vi "SetGlobalVariables.vi"   [LabVIEW 2023]
doc: "This VI sets non-robot specific constants and initializes critical global variables."
uses:
  GlobalMiscellaneous.vi
  GlobalDrivebase.vi
  GlobalPoseAndTargeting.vi
  GlobalShooter.vi
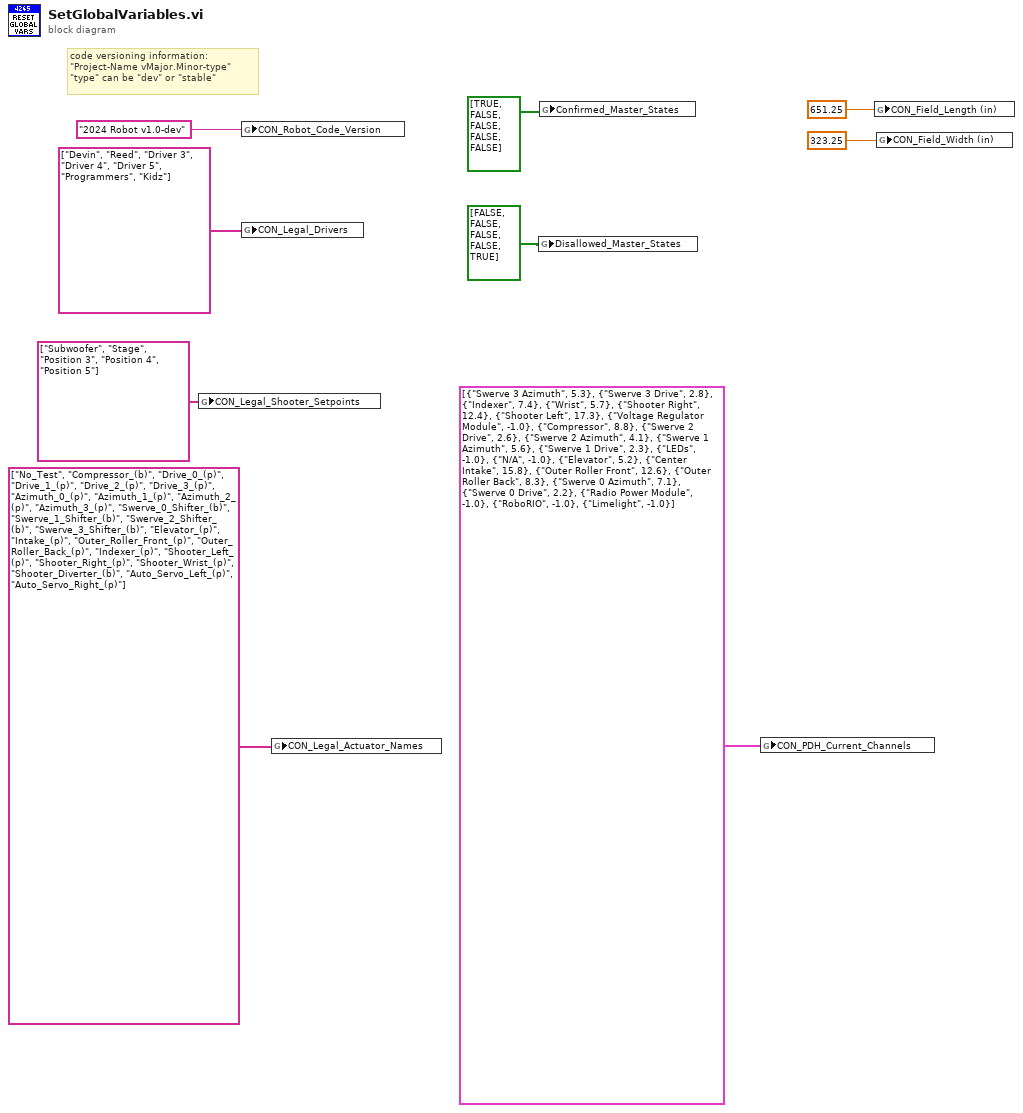
[diagram p0: block diagram]
diagram:
  # "code versioning information:\n\"Project-Name vMajor.Minor-type\"\n\"type\" can be \"dev\" or \"stable\""
  n1 = global write "GlobalShooter.vi" "CON_Legal_Shooter_Setpoints"(string[] ["Subwoofer", "Stage", "Position 3", "Position 4", "Position 5"] ("appended array")) -> ()
  n2 = global write "GlobalMiscellaneous.vi" "CON_Robot_Code_Version"("2024 Robot v1.0-dev" ("CON_Robot_Code_Version")) -> ()
  n3 = global write "GlobalDrivebase.vi" "CON_Legal_Drivers"(string[] ["Devin", "Reed", "Driver 3", "Driver 4", "Driver 5", "Programmers", "Kidz"] ("appended array")) -> ()
  n4 = global write "GlobalMiscellaneous.vi" "CON_Legal_Actuator_Names"(string[] ["No_Test", "Compressor_(b)", "Drive_0_(p)", "Drive_1_(p)", "Drive_2_(p)", "Drive_3_(p)", "Azimuth_0_(p)", "Azimuth_1_(p)", "Azimuth_2_(p)", "Azimuth_3_(p)", "Swerve_0_Shifter_(b)", "Swerve_1_Shifter_(b)", "Swerve_2_Shifter_(b)", "Swerve_3_Shifter_(b)", "Elevator_(p)", "Intake_(p)", "Outer_Roller_Front_(p)", "Outer_Roller_Back_(p)", "Indexer_(p)", "Shooter_Left_(p)", "Shooter_Right_(p)", "Shooter_Wrist_(p)", "Shooter_Diverter_(b)", "Auto_Servo_Left_(p)", "Auto_Servo_Right_(p)"] ("appended array")) -> ()
  n5 = global write "GlobalMiscellaneous.vi" "Disallowed_Master_States"(bool[] [FALSE, FALSE, FALSE, FALSE, TRUE] ("Disallowed_Master_States")) -> ()
  n6 = global write "GlobalMiscellaneous.vi" "Confirmed_Master_States"(bool[] [TRUE, FALSE, FALSE, FALSE, FALSE] ("Disallowed_Master_States")) -> ()
  n7 = global write "GlobalMiscellaneous.vi" "CON_PDH_Current_Channels"(cluster{string, dbl}[] [{"Swerve 3 Azimuth", 5.3}, {"Swerve 3 Drive", 2.8}, {"Indexer", 7.4}, {"Wrist", 5.7}, {"Shooter Right", 12.4}, {"Shooter Left", 17.3}, {"Voltage Regulator Module", -1.0}, {"Compressor", 8.8}, {"Swerve 2 Drive", 2.6}, {"Swerve 2 Azimuth", 4.1}, {"Swerve 1 Azimuth", 5.6}, {"Swerve 1 Drive", 2.3}, {"LEDs", -1.0}, {"N/A", -1.0}, {"Elevator", 5.2}, {"Center Intake", 15.8}, {"Outer Roller Front", 12.6}, {"Outer Roller Back", 8.3}, {"Swerve 0 Azimuth", 7.1}, {"Swerve 0 Drive", 2.2}, {"Radio Power Module", -1.0}, {"RoboRIO", -1.0}, {"Limelight", -1.0}]) -> ()
  n8 = global write "GlobalPoseAndTargeting.vi" "CON_Field_Length (in)"(651.25 ("CON_Field_Length (in)")) -> ()
  n9 = global write "GlobalPoseAndTargeting.vi" "CON_Field_Width (in)"(323.25 ("CON_Field_Length (in)")) -> ()
